vi "RD Digital In Trigger Set.vi"(8 "error in (no error)":errorcluster caption="错误输入（无错误）", 9 "Fall":u32, 10 "Rais":u32, 11 "handle":u64) -> (0 "error out":errorcluster caption="错误输出", 2 "function return":i32, 3 "handle out":u64)   [LabVIEW 2018, in "InstrumentsPlayground.lvlib"]
doc: "CLIFFAPI int CliffDigitalInTriggerSet(FT_HANDLE handle,uint Rais,uint Fall);\nwhen trigger mode == digital In trigger\nRais: for rasing trigger 0xFFFF as digtial IO IN 16->0 each switch\nFall: for falling trigger 0xFFFF as digtial IO IN 16->0 each switch\nyou can both enable or disable each ch's raising and falling trigger"
uses:
  InstrumentsPlayground.lvlib
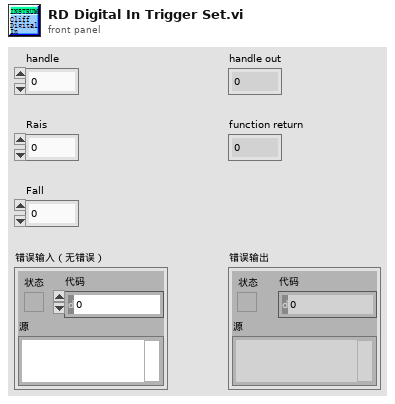
[diagram p1: front panel]
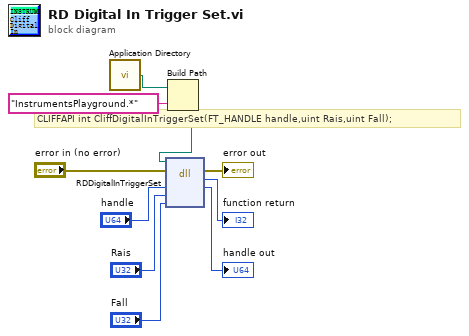
[diagram p0: block diagram]
diagram:
  # "CLIFFAPI int CliffDigitalInTriggerSet(FT_HANDLE handle,uint Rais,uint Fall);"
  n1 = call <vilib>:"Application Directory.vi"() -> ("Application Directory"=w2:path)
  n2 = Build Path(base path=w2, name or relative path="InstrumentsPlayground.*" ("名称或相对路径")) -> (appended path=w1:path)
  n3 = dll-call lib="E:/work/YZCourse_Xtext/Cliff/API/LabVIEW lib/InstrumentsPlayground.*" fn="RDDigitalInTriggerSet"(path in=w1, error in="error in (no error)", "handle"="handle", "Rais"="Rais", "Fall"="Fall") -> (error out=→"error out":errorcluster, "返回类型"=→"function return":i32, "handle"=→"handle out":u64)  [unwired: 3 in, 1 out]
